vi "TestBed_Headers.vi"() -> ()   [LabVIEW 2018]
doc: "<b> </b> <b> </b>\nHttpClient_NET\nJustin Young - Viviota\nCopyright (c) 2021\nLicense: BSD"
uses:
  HttpHeaders_Request/HttpHeaders_Request.lvclass
  C:/Viviota/Projects/R&D/__OpenSource/VIV_HTTP_REST_NET/HTTPHeaders_NET/HttpHeaders_NET.lvclass
  System.Net.Http
  HTTPHeaders_NET/HttpHeaders_NET.lvclass
panel:
  out "Header Names 2":string[](array[string])
  out "Header Values 2":string[](array[string])
  out "Header Values":string[](array[string])
  out "Header Names":string[](array[string])
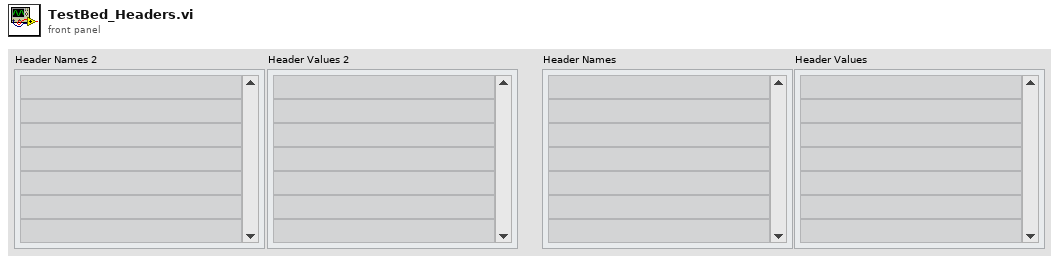
[diagram p1: front panel]
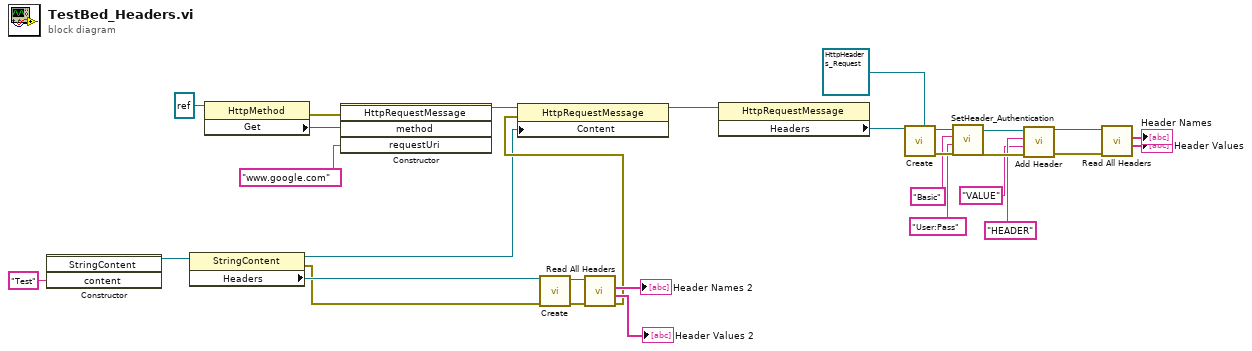
[diagram p0: block diagram]
diagram:
  n1 = constructor class="StringContent"("content"="Test") -> (reference out=w27:refnum<k24>)  [unwired: 3 in, 3 out]
  n2 = property class="StringContent"(reference=w27) -> (reference out=w9:refnum<k24>, error out=w17:errorcluster, "Headers"=w25:refnum<k24>)  [unwired: 1 in]
  n3 = property class="HttpMethod"(reference=refnum<k24> refnum) -> (error out=w29:errorcluster, "Get"=w23:refnum<k24>)  [unwired: 1 in, 1 out]
  n4 = constructor class="HttpRequestMessage"(error in=w29, "method"=w23, "requestUri"="www.google.com") -> (reference out=w28:refnum<k24>)  [unwired: 2 in, 4 out]
  n5 = call "Create.vi"("error in (no error)"=w17, "NET_HttpHeaders"=w25) -> ("error out"=w16:errorcluster, "HTTPHeaders_NET out"=w1:refnum<class "HttpHeaders_NET.lvclass">)  [unwired: 8 in]
  n6 = call-dynamic "Read All Headers.vi"("error in (no error)"=w16, "HTTPHeaders_NET in"=w1) -> ("error out"=w15:errorcluster, "Header Values"=→"Header Values 2":string[], "Header Names"=→"Header Names 2":string[])  [unwired: 6 in, 1 out]
  n7 = property class="HttpRequestMessage"(reference=w28, error in=w15, "Content"=w9) -> (reference out=w24:refnum<k24>)  [unwired: 1 out]
  n8 = property class="HttpRequestMessage"(reference=w24) -> ("Headers"=w2:refnum<k24>)  [unwired: 1 in, 2 out]
  n9 = call "Create.vi"("HTTPHeaders_NET in"=refnum<class "HttpHeaders_Request.lvclass"> refnum ("LabVIEWHTTPClient_NET.lvlib:HttpHeaders_Request.lvclass"), "NET_HttpHeaders"=w2) -> ("error out"=w12:errorcluster, "HTTPHeaders_NET out"=w13:refnum<class "HttpHeaders_Request.lvclass">)  [unwired: 8 in]
  n10 = call "SetHeader_Authentication.vi"("error in (no error)"=w12, "parameter"="User:Pass", "scheme"="Basic", "HttpHeaders_Request in"=w13) -> ("error out"=w7:errorcluster, "HttpHeaders_Request out"=w8:refnum<class "HttpHeaders_Request.lvclass">)  [unwired: 6 in]
  n11 = call-dynamic "Add Header.vi"("error in (no error)"=w7, "Value"="VALUE", "Name"="HEADER", "HTTPHeaders_NET in"=w8) -> ("error out"=w5:errorcluster, "HTTPHeaders_NET out"=w6:refnum<class "HttpHeaders_Request.lvclass">)  [unwired: 6 in]
  n12 = call-dynamic "Read All Headers.vi"("error in (no error)"=w5, "HTTPHeaders_NET in"=w6) -> ("Header Values"=→"Header Values":string[], "Header Names"=→"Header Names":string[])  [unwired: 6 in, 2 out]
